vi "PID simulation.vi"() -> ()   [LabVIEW 2011]
uses:
  <vilib>/addons/control/pid/pid.llb/PID (DBL).vi
  <vilib>/Analysis/coordinate.llb/2D Cartesian Coordinate Rotation (Scalar).vi
  <vilib>/Analysis/NI_AALPro.lvlib
  <vilib>/addons/control/pid/NI_PID_pid.lvlib
panel:
  in  "milliseconds to wait":u32
  out "X current":dbl
  out "Y current":dbl
  in  "stop":bool
  out "Y speed":dbl
  out "X speed":dbl
  in  "Y rate":dbl
  in  "X rate":dbl
  in  "Y-Start":dbl
  in  "X-Start":dbl
  in  "Speed":dbl
  in  "Ramp":dbl
  in  "Y-Goal":dbl
  in  "X-Goal":dbl
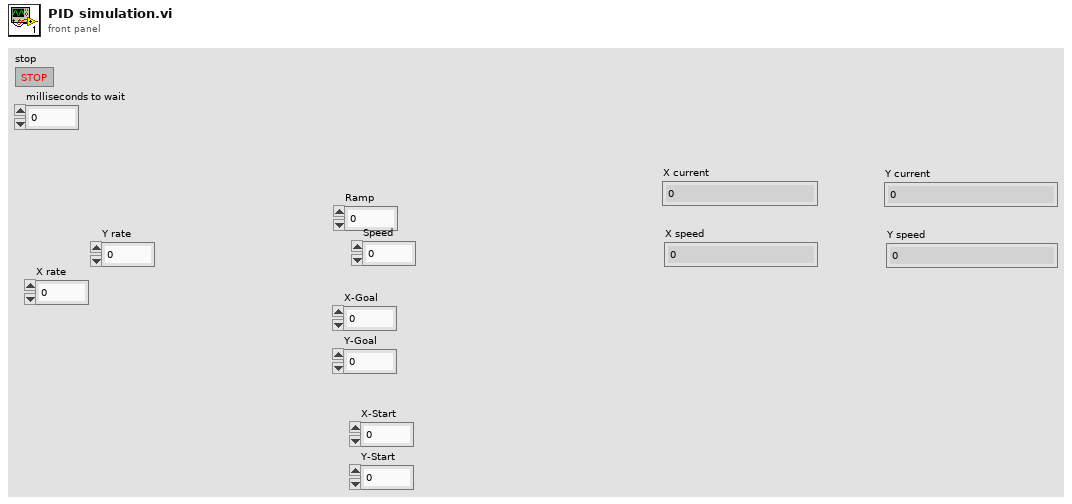
[diagram p1: front panel]
types:
  T1 = cluster{"proportional gain (Kc)":dbl, "integral time (Ti, min)":dbl, "derivative time (Td, min)":dbl}
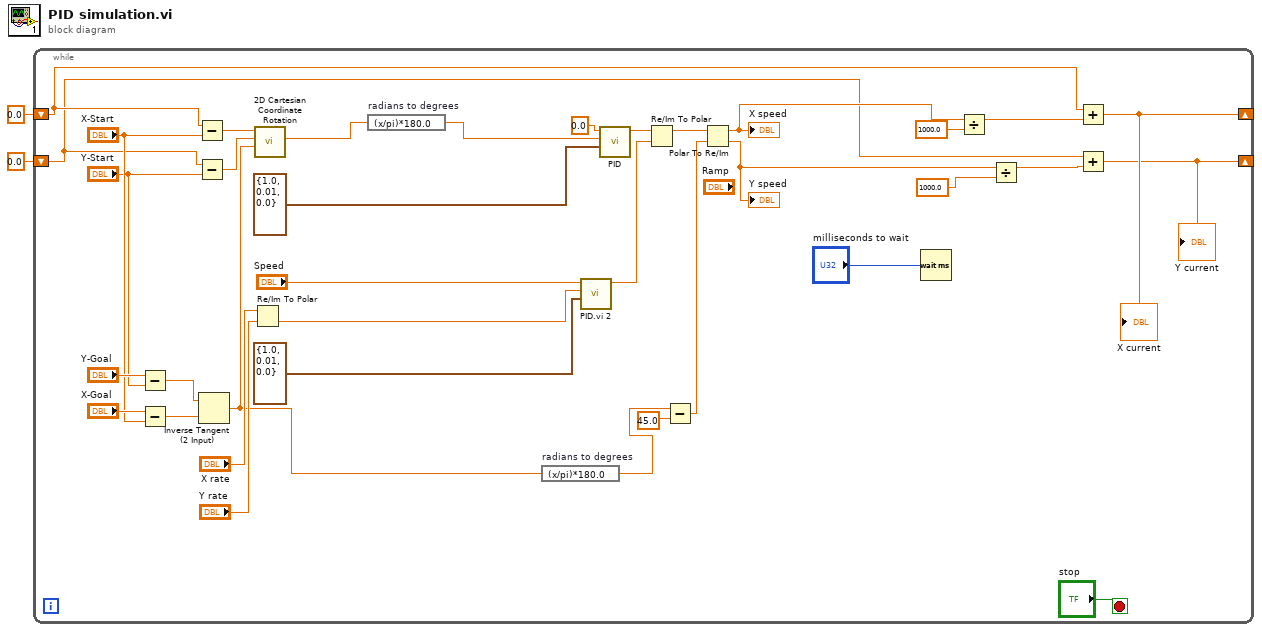
[diagram p0: block diagram]
diagram:
  n1 = while {
    shift-right: [w15] -> _
    shift-left: 0.0 -> [w11]
    shift-right: [w14] -> _
    shift-left: 0.0 -> [w10]
    stop <- "stop" stop-if-true
    n2 = Subtract(x="Y-Goal", y="Y-Start") -> (x-y=w33:dbl)
    n3 = Subtract(x="X-Goal", y="X-Start") -> (x-y=w34:dbl)
    n4 = Subtract(x=w11, y="X-Start") -> (x-y=w32:dbl)
    n5 = Subtract(x=w10, y="Y-Start") -> (x-y=w31:dbl)
    n6 = Inverse Tangent (2 Input)(1:w34, 2:w33) -> (0:w17:dbl)
    n7 = Re/Im To Polar(2:"Y rate", 3:"X rate") -> (0:w20:dbl)  [unwired: 1 out]
    n8 = call-poly <vilib>:"2D Cartesian Coordinate Rotation.vi"("theta"=w17, "y"=w31, "x"=w32) -> ("y out"=w9:dbl)  [unwired: 6 in, 2 out]
    n9 = expression code="(x/pi)*180.0" "radians to degrees"(w9) -> (w8:dbl)
    n10 = expression code="(x/pi)*180.0" "radians to degrees"(w17) -> (w16:dbl)
    n11 = call-poly "PID.vi 2"("PID gains"=T1 {"proportional gain (Kc)"=1.0, "integral time (Ti, min)"=0.01, "derivative time (Td, min)"=0.0}, "process variable"=w20, "setpoint"="Speed") -> ("output"=w21:dbl)  [unwired: 7 in, 1 out]
    n12 = call-poly <vilib>:"PID.vi"("PID gains"=T1 {"proportional gain (Kc)"=1.0, "integral time (Ti, min)"=0.01, "derivative time (Td, min)"=0.0}, "process variable"=w8, "setpoint"=0.0) -> ("output"=w24:dbl)  [unwired: 7 in, 1 out]
    n13 = Re/Im To Polar(2:w21, 3:w24) -> (1:w26:dbl)  [unwired: 1 out]
    n14 = Subtract(x=w16, y=45.0) -> (x-y=w27:dbl)
    n15 = Polar To Re/Im(2:w27, 3:w26) -> (0:w12:dbl, 1:w13:dbl)
    "X speed" <- w13
    "Y speed" <- w12
    n16 = Wait (ms)(milliseconds to wait="milliseconds to wait") -> ()  [unwired: 1 out]
    n17 = Divide(x=w13, y=1000.0) -> (x/y=w7:dbl)
    n18 = Divide(x=w12, y=1000.0) -> (x/y=w4:dbl)
    n19 = Add(x=w11, y=w7) -> (x+y=w15:dbl)
    "X current" <- w15
    n20 = Add(x=w10, y=w4) -> (x+y=w14:dbl)
    "Y current" <- w14
  }
